vi "FlatToRichnixnet_grpc_FutureTimeTriggerRequest.vi"(5 "OutputClusterType":T1, 11 "InputCluster":T3) -> (3 "OutputCluster":T1)   [LabVIEW 2025, in "xnet-grpc_client.lvlib"]
uses:
  nixnet_grpc_FutureTimeTriggerRequest_Flat.ctl
  nidevice_grpc_Session_Flat.ctl
  nixnet_grpc_TimeScale.ctl
  nixnet_grpc_FutureTimeTriggerRequest.ctl
  nixnet_grpc_FutureTimeTriggerRequest_timescale_enum/nixnet_grpc_FutureTimeTriggerRequest_timescale_enum.lvclass
  nidevice_grpc_Session.ctl
  xnet-grpc_client.lvlib
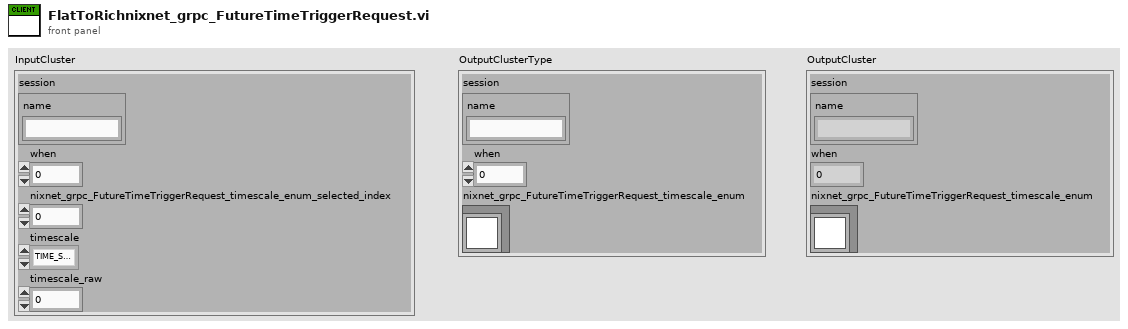
[diagram p1: front panel]
types:
  T1 = typedef "xnet-grpc_client.lvlib/nixnet_grpc_FutureTimeTriggerRequest.ctl" = cluster{"session":T2, "when":u64, "nixnet_grpc_FutureTimeTriggerRequest_timescale_enum":refnum<class "nixnet_grpc_FutureTimeTriggerRequest_timescale_enum.lvclass">}
  T2 = typedef "xnet-grpc_client.lvlib/nidevice_grpc_Session.ctl" = cluster{"name":string}
  T3 = typedef "xnet-grpc_client.lvlib/nixnet_grpc_FutureTimeTriggerRequest_Flat.ctl" = cluster{"session":T4, "when":u64, "nixnet_grpc_FutureTimeTriggerRequest_timescale_enum_selected_index":i32, "timescale":T5, "timescale_raw":u32}
  T4 = typedef "xnet-grpc_client.lvlib/nidevice_grpc_Session_Flat.ctl" = cluster{"name":string}
  T5 = typedef "xnet-grpc_client.lvlib/nixnet_grpc_TimeScale.ctl" = enum32{"TIME_SCALE_LOCAL_TIME", "TIME_SCALE_NETWORK_TIME"}
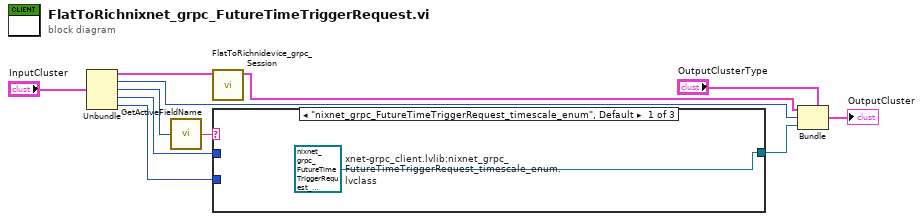
[diagram p0: block diagram]
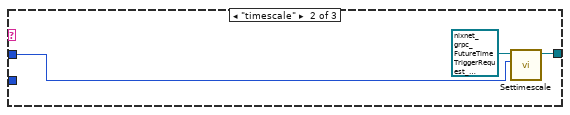
[diagram p2: hidden frame]
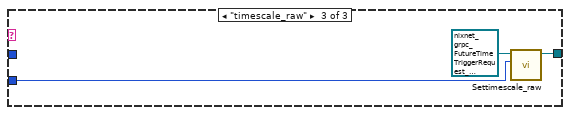
[diagram p3: hidden frame]
diagram:
  n1 = Unbundle "Unbundle"("InputCluster") -> ("session"=w8:T4, "when"=w6:u64, "nixnet_grpc_FutureTimeTriggerRequest_timescale_enum_selected_index"=w5:i32, "timescale"=w2:T5, "timescale_raw"=w1:u32)
  n2 = call "GetActiveFieldName.vi"("protobuf index"=w5) -> ("oneof field name"=w4:string)
  n3 = call "FlatToRichnidevice_grpc_Session.vi"("InputCluster"=w8) -> ("OutputCluster"=w7:T2)  [unwired: 10 in]
  n4 = case "nixnet_grpc_FutureTimeTriggerRequest_timescale_enum" shown="\"nixnet_grpc_FutureTimeTriggerRequest_timescale_enum\", Default" w4 {
    tunnel: [w12 w14 w17] -> w3
    tunnel: w2 -> [_ w15 _]
    tunnel: w1 -> [_ _ w18]
    frame "nixnet_grpc_FutureTimeTriggerRequest_timescale_enum", Default {
      w12 = refnum<class "nixnet_grpc_FutureTimeTriggerRequest_timescale_enum.lvclass"> refnum  # xnet-grpc_client.lvlib:nixnet_grpc_FutureTimeTriggerRequest_timescale_enum.lvclass
    }
    frame "timescale" {
      n5 = call "Settimescale.vi"("Set_Val"=w15, "OneOfTemplate in"=refnum<class "nixnet_grpc_FutureTimeTriggerRequest_timescale_enum.lvclass"> refnum) -> ("OneOfTemplate out"=w14:refnum<class "nixnet_grpc_FutureTimeTriggerRequest_timescale_enum.lvclass">)  [unwired: 8 in, 1 out]
    }
    frame "timescale_raw" {
      n6 = call "Settimescale_raw.vi"("Set_Val"=w18, "OneOfTemplate in"=refnum<class "nixnet_grpc_FutureTimeTriggerRequest_timescale_enum.lvclass"> refnum) -> ("OneOfTemplate out"=w17:refnum<class "nixnet_grpc_FutureTimeTriggerRequest_timescale_enum.lvclass">)  [unwired: 8 in, 1 out]
    }
  }
  n7 = Bundle "Bundle"(cluster="OutputClusterType", "session"=w7, "when"=w6, "nixnet_grpc_FutureTimeTriggerRequest_timescale_enum"=w3) -> (→"OutputCluster":T1)
